vi "Timeout.vi"(8 "error in (no error)":errorcluster, 10 "Data":variant, 11 "Storage in":refnum<class "Storage.lvclass">) -> (0 "error out":errorcluster, 3 "Storage out":refnum<class "Storage.lvclass">)   [LabVIEW 2015, in "AMS UI.lvlib" / "Storage.lvclass"]
uses:
  Storage.lvclass
  AMS Gas Actor/AMS Gas Actor.lvclass
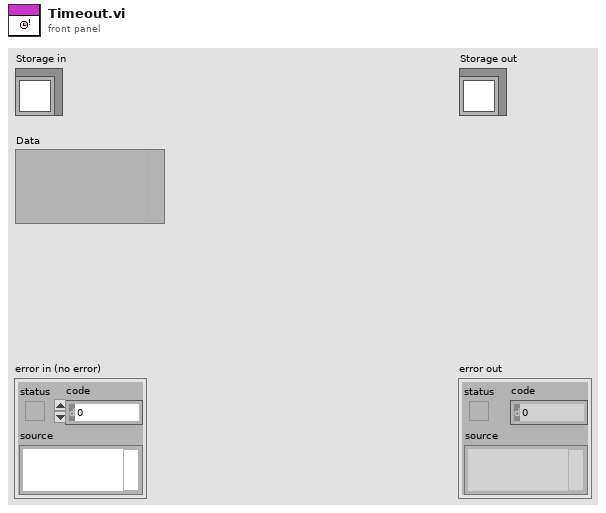
[diagram p1: front panel]
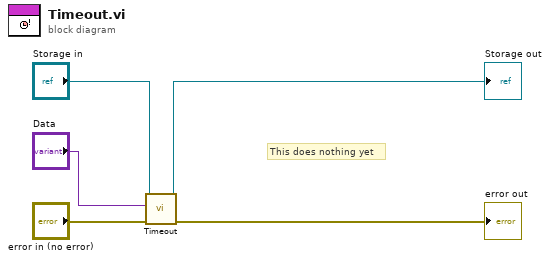
[diagram p0: block diagram]
diagram:
  # "This does nothing yet"
  n1 = call-parent "Timeout.vi"("error in (no error)"="error in (no error)", "Data"="Data", "eActor in"="Storage in") -> ("error out"=→"error out":errorcluster, "eActor out"=→"Storage out":refnum<class "Storage.lvclass">)  [unwired: 7 in]
